vi "Read Common Config.vi"(8 "error in (no error)":errorcluster, 11 "CIFTemplateNode in":refnum<class "CIFTemplateNode.lvclass">) -> (0 "error out":errorcluster, 2 "Common":T1={"Period (s)"=0.001, "T0 (ns)"=0, "ClockID"=0, "Priority"=100, "Processor"=-2} {"Period (s)" format="%#_13g"}, 3 "CIFTemplateNode out":refnum<class "CIFTemplateNode.lvclass">)   [LabVIEW 2021, in "CIFTemplateNode.lvclass"]
uses:
  CIFTemplateNode.lvclass
  CIFTemplateNode.lvclass/CIFTemplateNode.ctl
  CIFTemplateCommon/Typedef/Common Plugin Configuration.ctl
  CIFTemplateCommon/CIFTemplateCommon.lvlib
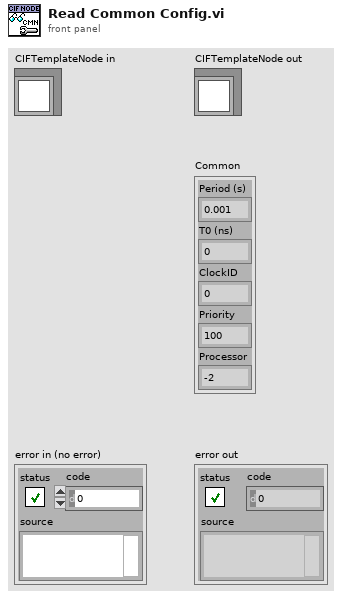
[diagram p1: front panel]
types:
  T1 = typedef "CIFTemplateCommon.lvlib/Common Plugin Configuration.ctl" = cluster{"Period (s)":dbl, "T0 (ns)":u64, "ClockID":u8, "Priority":i32, "Processor":i32}
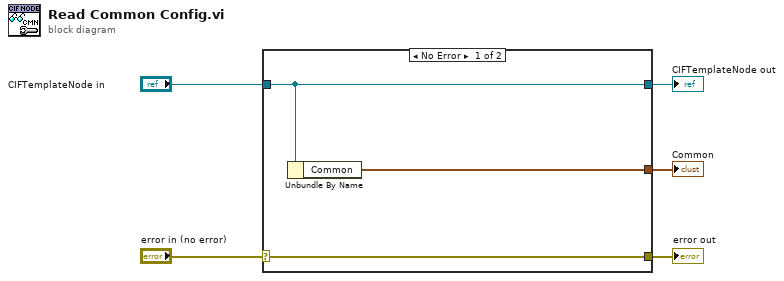
[diagram p0: block diagram]
diagram:
  n1 = case shown="No Error" "error in (no error)" {
    selector: "error in (no error)" -> [w8 w9]
    tunnel: [w8 w9] -> w4
    tunnel: [w7 w10] -> w2
    tunnel: "CIFTemplateNode in" -> [w7 w10]
    tunnel: [w6 _] -> w1
    frame No Error {
      n2 = Unbundle By Name(w7) -> ("Common"=w6:T1)
    }
    frame Error {
    }
  }
  "error out" <- w4
  "CIFTemplateNode out" <- w2
  "Common" <- w1
